vi "direct_abs_con_p_XT.vi"(0 "WorkingPair (Input)":T1={"no_iso"=1, "no_p_sat"=1, "path_db"="D:\\Driesel\\SorpLibLocal\\LabVIEW_wrapper\\data\\json\\sorpproplib_minimalExample.json", "wp_as"="silicagel", "wp_st"="123", "wp_iso"="DubininArctan1", "wp_rf"="water", "rf_rhol"="SaturatedLiquidDensity_EoS1", "no_rhol"=1, "rf_psat"="VaporPressure_EoS1"}, 5 "Concentration in kg/kg (Input)":dbl, 7 "Temperature in K (Input)":dbl, 11 "Error (Input)":errorcluster) -> (4 "Pressure in Pa (Output)":dbl, 15 "Error (Output)":errorcluster)   [LabVIEW 2017]
doc: "direct_abs_con_p_XT:\n * --------------------\n *\n * Calculates equilibrium pressure p in Pa depending on equilibrium\n * concentration X in kg/kg and equilibrium temperature T in K.\n *\n * Parameters:\n * -----------\n * double X_kgkg:\n * Equilibrium concentration in kg/kg.\n * double T_K:\n * Equilibrium temperature in K.\n *\n * const char *path_db:\n * Path to database.\n * const char *wp_as:\n * Name of sorbent.\n * const char *wp_st:\n * Name of sub-type of sorbent.\n * const char *wp_rf:\n * Name of refrigerant.\n * const char *wp_iso:\n * Name of isotherm.\n * int no_iso:\n * ID of isotherm (i.e. when more than one isotherm is available)\n * const char *rf_psat:\n * Name of calculation approach for vapor pressure.\n * int no_p_sat:\n * ID of vapor pressure equation (i.e. when more than one equation is\n * available)\n * const char *rf_rhol:\n * Name of calculation approach for liquid density.\n * int no_rhol:\n * ID of liquid density equation (i.e. when more than one equation is\n * available)\n *\n * Returns:\n * --------\n * double:\n * Equilibrium pressure in Pa.\n *\n * Remarks:\n * --------\n * This function is only valid for isotherm models based on the conventional\n * approach.\n *\n * History:\n * --------\n * 07/12/2020, by Jannik Driesel (supervised by Mirko Engelpracht):\n * First implementation."
uses:
  data/win32bit/libsorpPropLib.dll
panel:
  # "Path to database"
  # "Name of sorbent"
  # "Name of sub-type of sorbent"
  # "Name of refrigerant"
  # "Name of isotherm"
  # "ID of isotherm"
  # "Name of calculation approach for vapor pressure"
  # "ID of vapor pressure equation"
  # "Name of calculation approach for liquid density"
  # "ID of liquid density equation"
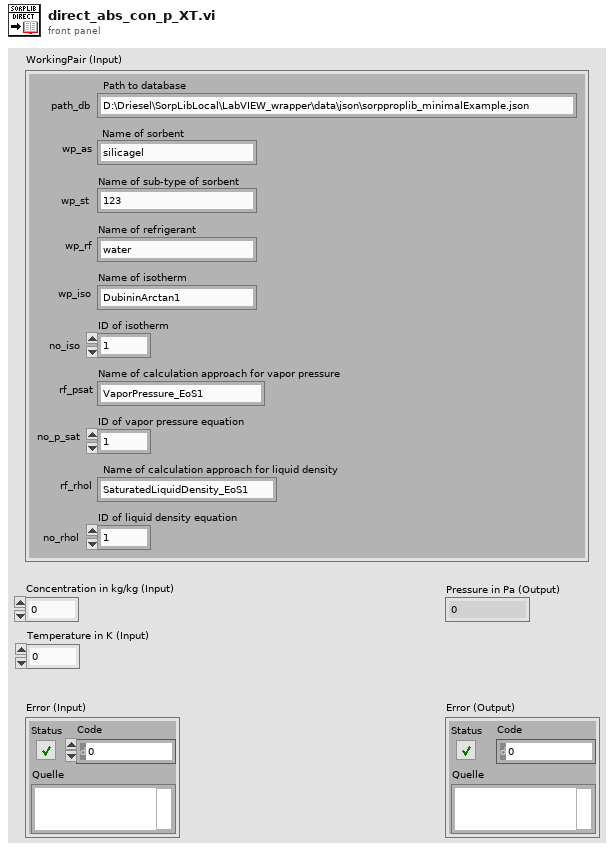
[diagram p1: front panel]
types:
  T1 = cluster{"no_iso":i32, "no_p_sat":i32, "path_db":string, "wp_as":string, "wp_st":string, "wp_iso":string, "wp_rf":string, "rf_rhol":string, "no_rhol":i32, "rf_psat":string}
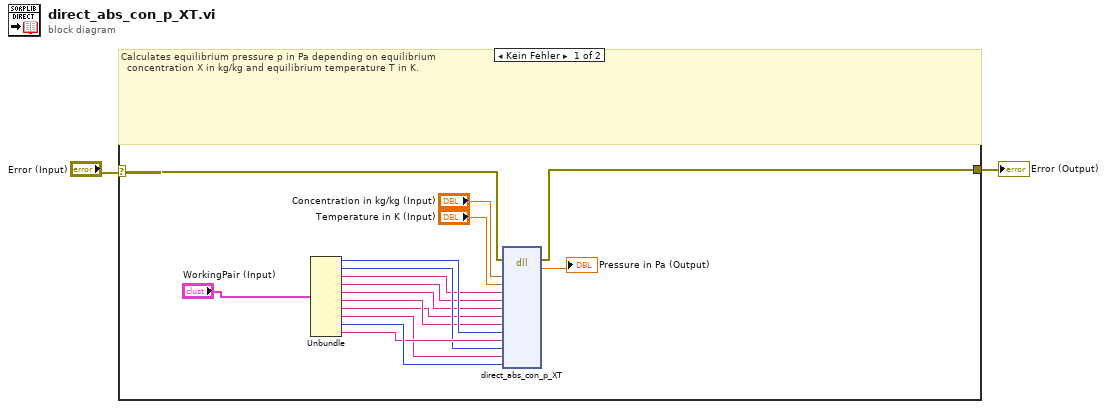
[diagram p0: block diagram]
diagram:
  n1 = case shown="Kein Fehler" "Error (Input)" {
    selector: "Error (Input)" -> [w8 w19]
    tunnel: [w7 w19] -> w2
    frame No Error {
      # "Calculates equilibrium pressure p in Pa depending on equilibrium\n  concentration X in kg/kg and equilibrium temperature T in K."
      n2 = Unbundle("WorkingPair (Input)") -> ("no_iso"=w15:i32, "no_p_sat"=w16:i32, "path_db"=w9:string, "wp_as"=w10:string, "wp_st"=w11:string, "wp_iso"=w13:string, "wp_rf"=w12:string, "rf_rhol"=w14:string, "no_rhol"=w18:i32, "rf_psat"=w17:string)
      n3 = dll-call lib="D:/Driesel/SorpLibLocal/LabVIEW_wrapper/data/win32bit/libsorpPropLib.dll" fn="direct_abs_con_p_XT"(error in=w8, "X_kgkg"="Concentration in kg/kg (Input)", "T_K"="Temperature in K (Input)", "path_db"=w9, "wp_as"=w10, "wp_st"=w11, "wp_rf"=w12, "wp_iso"=w13, "no_iso"=w15, "rf_psat"=w17, "no_p_sat"=w16, "rf_rhol"=w14, "no_rhol"=w18) -> (error out=w7:errorcluster, "p_Pa"=→"Pressure in Pa (Output)":dbl)  [unwired: 14 in, 1 out]
    }
    frame Error {
      # "Error - No calculations"
    }
  }
  "Error (Output)" <- w2
